vi "DrawPoint.vi"(4 "Pen":refnum<class "Pen.lvclass">=refnum, 6 "Color":refnum<class "Color.lvclass">=refnum, 8 "error in (no error)":errorcluster, 10 "Point":refnum<class "Point.lvclass">=refnum, 11 "picture in":picture) -> (0 "error out":errorcluster, 3 "picture out":picture)   [LabVIEW 2020, in "2DPictureControl.lvclass"]
uses:
  2DPictureControl.lvclass
  Point/Point.lvclass
  Pen/Pen.lvclass
  Color/Color.lvclass
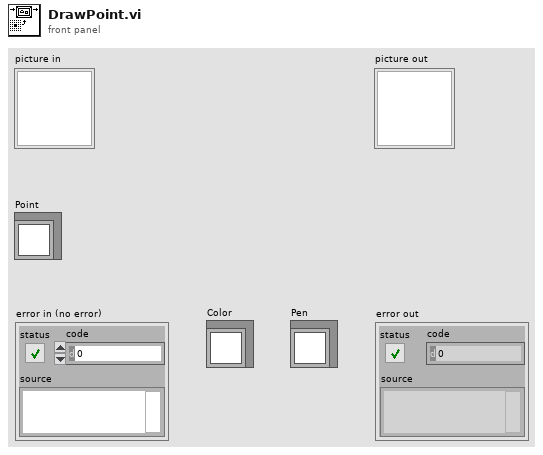
[diagram p1: front panel]
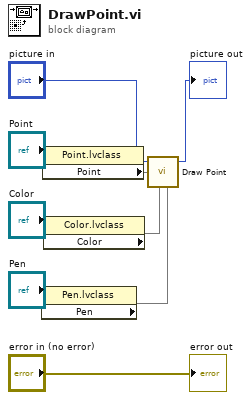
[diagram p0: block diagram]
diagram:
  n1 = property class="Pen.lvclass"(reference="Pen") -> ("Pen"=w4)  [unwired: 1 in, 2 out]
  n2 = property class="Point.lvclass"(reference="Point") -> ("Point"=w6)  [unwired: 1 in, 2 out]
  n3 = property class="Color.lvclass"(reference="Color") -> ("Color"=w1)  [unwired: 1 in, 2 out]
  n4 = call <vilib>:"Draw Point.vi"("picture"="picture in", "point(x,y)"=w6, "color(black)"=w1, "pen"=w4) -> ("new picture"=→"picture out":picture)  [unwired: 5 in]
  "error out" <- "error in (no error)"
